vi "pfz1.vi"(8 "R(k-2)":dbl, 9 "R(k-1)":dbl, 10 "U(k-2)":dbl) -> (2 "R(k)":dbl)   [LabVIEW 2019]
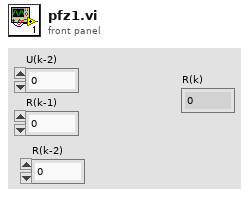
[diagram p1: front panel]
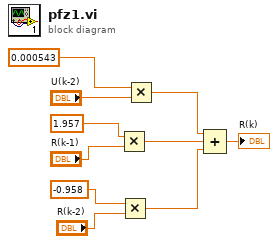
[diagram p0: block diagram]
diagram:
  n1 = Multiply(x=1.957, y="R(k-1)") -> (x*y=w3:dbl)
  n2 = Multiply(x=-0.958, y="R(k-2)") -> (x*y=w1:dbl)
  n3 = Multiply(x=0.000543, y="U(k-2)") -> (x*y=w2:dbl)
  n4 = Compound Arithmetic op=ADD(w2, w3, w1) -> (→"R(k)":dbl)
